vi "Process Button Pressed.vi"(8 "error in (no error)":errorcluster, 10 "Menu Reference":refnum<vi>, 11 "MenuButton Event Handler in":refnum<class "MenuButton Event Handler.lvclass">) -> (0 "error out":errorcluster, 3 "MenuButton Event Handler out":refnum<class "MenuButton Event Handler.lvclass">)   [LabVIEW 2017, in "MenuButtons.lvlib" / "MenuButton Event Handler.lvclass"]
uses:
  MenuButton Event Handler.lvclass
  MenuButton Event Handler.lvclass/MenuButton Event Handler.ctl
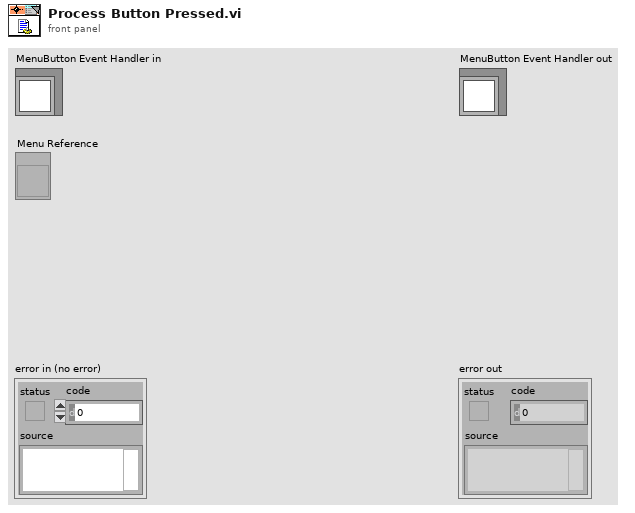
[diagram p1: front panel]
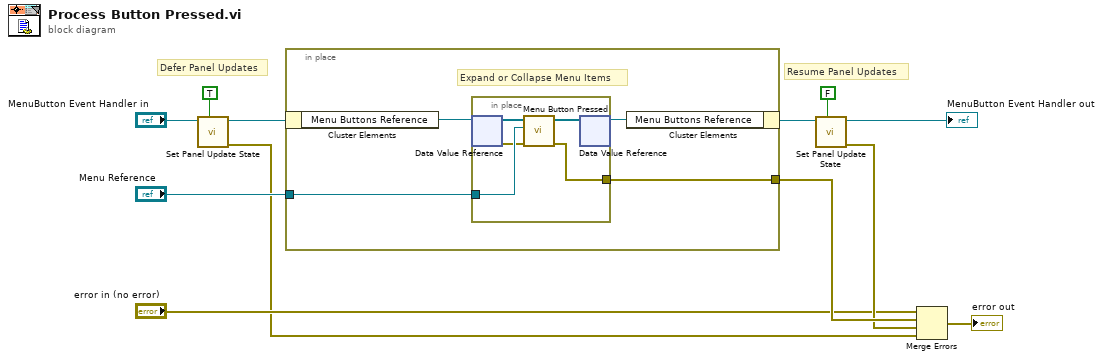
[diagram p0: block diagram]
diagram:
  # "Resume Panel Updates"
  # "Defer Panel Updates"
  n1 = call "Set Panel Update State.vi"("Defer?"=TRUE, "MenuButton Event Handler in"="MenuButton Event Handler in") -> ("error out"=w1:errorcluster, "MenuButton Event Handler out"=w9:refnum<class "MenuButton Event Handler.lvclass">)  [unwired: 8 in]
  n2 = in-place {
    in-place-border: "Menu Reference" -> [w16]
    in-place-border: [w13] -> w5
    # "Expand or Collapse Menu Items"
    n3 = in-place-cluster #1(w9) -> ("Menu Buttons Reference"=w15:refnum<data-value>)
    n4 = in-place {
      in-place-border: w16 -> [w21]
      in-place-border: [w17] -> w13
      n5 = in-place-dvr #2(w15) -> (w20:refnum<class "MenuButton.lvclass">[], w18:errorcluster)
      n6 = call "Menu Button Pressed.vi"("error in (no error)"=w18, "Menu Reference"=w21, "Menu Items In"=w20) -> ("error out"=w17:errorcluster, "Menu Items Out"=w19:refnum<class "MenuButton.lvclass">[])  [unwired: 7 in]
      n7 = in-place-dvr #2(w19) -> (w14:refnum<data-value>)  [unwired: 1 out]
    }
    n8 = in-place-cluster #1("Menu Buttons Reference"=w14) -> (w7:refnum<class "MenuButton Event Handler.lvclass">)
  }
  n9 = call "Set Panel Update State.vi"("Defer?"=FALSE, "MenuButton Event Handler in"=w7) -> ("error out"=w4:errorcluster, "MenuButton Event Handler out"=→"MenuButton Event Handler out":refnum<class "MenuButton Event Handler.lvclass">)  [unwired: 8 in]
  n10 = Merge Errors("error in (no error)", w5, w4, w1) -> (→"error out":errorcluster)
